vi "Dashboard Main.vi"() -> ()   [LabVIEW 2017]
uses:
  Common Code/Drivetrain Status Cluster.ctl
  Common Code/Drivetrain Mode.ctl
  Common Code/DT Encoder Values.ctl
  Common Code/Intake Status Cluster.ctl
  Common Code/Intake Mode.ctl
  Common Code/Intake States.ctl
  Common Code/Elevator Status Cluster.ctl
  Common Code/Elevator State.ctl
  Common Code/Elevator Mode.ctl
  Common Code/Intake PDP Info.ctl
  Common Code/Intake Presets.ctl
  Common Code/Drivetrain Settings Cluster.ctl
  Common Code/PID Gains Cluster.ctl
  Common Code/Elevator Settings Cluster.ctl
  Common Code/PID Gains.ctl
  Common Code/Climb Status Cluster.ctl
  Common Code/Dashboard Control Data.ctl
  Common Code/Robot Name.ctl
  Common Code/Dashboard Status Data.ctl
  <vilib>/Rock Robotics/WPI/Dashboard/WPI_DashboardLogging Global.vi
  <vilib>/Utility/inputDevices.llb/keyboardAcquire.vi
  Robot Code/Robot Global Data.vi
panel:
  in  "Save":bool
  in  "Load":bool
  out "DumbDashMessage":string
  in  "stop":bool
  in  "Tab Control":T1(tab)
  in  "Robot IP":string
  out "Drivetrain Status Cluster":T2 {"Gyro" scale=-180.0..180.0}
  in  "Drivetrain Settings Cluster":T5
  out "Elevator Status Cluster":T7={"Finished"=FALSE, "Elevator Power"=0.0, "Elevator State"=enum."Idle", "Elevator Mode"=enum."Manual", "Elevator Height"=0.0, "At Bottom?"=FALSE, "At Top?"=FALSE, "Scale high?"=FALSE, "PID Output"=0.0}
  in  "Elevator Settings Cluster":T10={"Ground Height"=0.0, "Switch Height"=0.0, "Scale High Height "=0.0, "Scale Low Height"=0.0, "Elevator PID Gains"={"proportional gain (Kc)"=1.0, "integral time (Ti, min)"=0.01, "derivative time (Td, min)"=0.0}, "Elevator Tolerance"=0.0, "Reset Encoders"=FALSE, "Encoder Scale"=0.0, "Max Height"=0.0, "Mid Height"=0.0, "output range"={"output high"=100.0, "output low"=-100.0}} {"Elevator PID Gains"."derivative time (Td, min)" format="%.3f"; "Elevator PID Gains"."integral time (Ti, min)" format="%.3f"; "Elevator PID Gains"."proportional gain (Kc)" format="%.3f"}
  out "Intake PDP Info":T12
  out "Intake Status Cluster":T13={"Intake Mode"=enum."Manual", "Intake States"=enum."Zero", "Intake Current Angle"=0.0, "Cube In Posession?"=FALSE, "Intake Wrist Up?"=FALSE}
  in  "Intake Presets":T16={"Idle Angle"=0.0, "Mid Angle"=0.0, "Low Angle"=0.0, "Outtake Power"=0.0, "Intake Power"=0.0, "Unstuck"=0.0, "Angle Tolerance"=0.0, "Max Angle"=0.0, "Max Current"=0.0, "Current Trip Time"=0.0, "Reset Encoder?"=FALSE, "Encoder Scale"=0.0, "PID gains"={"proportional gain (Kc)"=0.0, "integral time (Ti, min)"=0.0, "derivative time (Td, min)"=0.0}, "output range"={"output high"=100.0, "output low"=-100.0}}
  out "Climb Status Cluster":T17
  in  "TCP":refnum<k5>
  in  "Rec Mode":enum32{"Stop", "Record", "Playback"}(radio)
  # "A2"
  # "A3"
  # "Driver :\n\nA1 - \nA2 -\nA3 - \nA4 - \nA5 - \nB0 - \nB1 -\nB2 -\nB3 -\nB4 -\nB5 -\nB6 -\nB7 -\nB8 -\nB9 -\nUp -\nDown - \nLeft -\nRight -"
  # "Manipulator :\n\nA1 -  \nA2 -\nA3 - \nA4 - \nA5 - \nB0 - \nB1 -\nB2 -\nB3 -\nB4 -\nB5 -\nB6 -\nB7 -\nB8 -\nB9 - \nUp -\nDown - \nLeft -\nRight -"
  # "B4"
  # "B5"
  # "B6"
  # "B7"
  # "B3"
  # "U"
  # "B2"
  # "B1"
  # "L"
  # "R"
  # "A5"
  # "A1"
  # "B0"
  # "D"
  # "A0"
  # "A4"
  # "B8"
  # "B9"
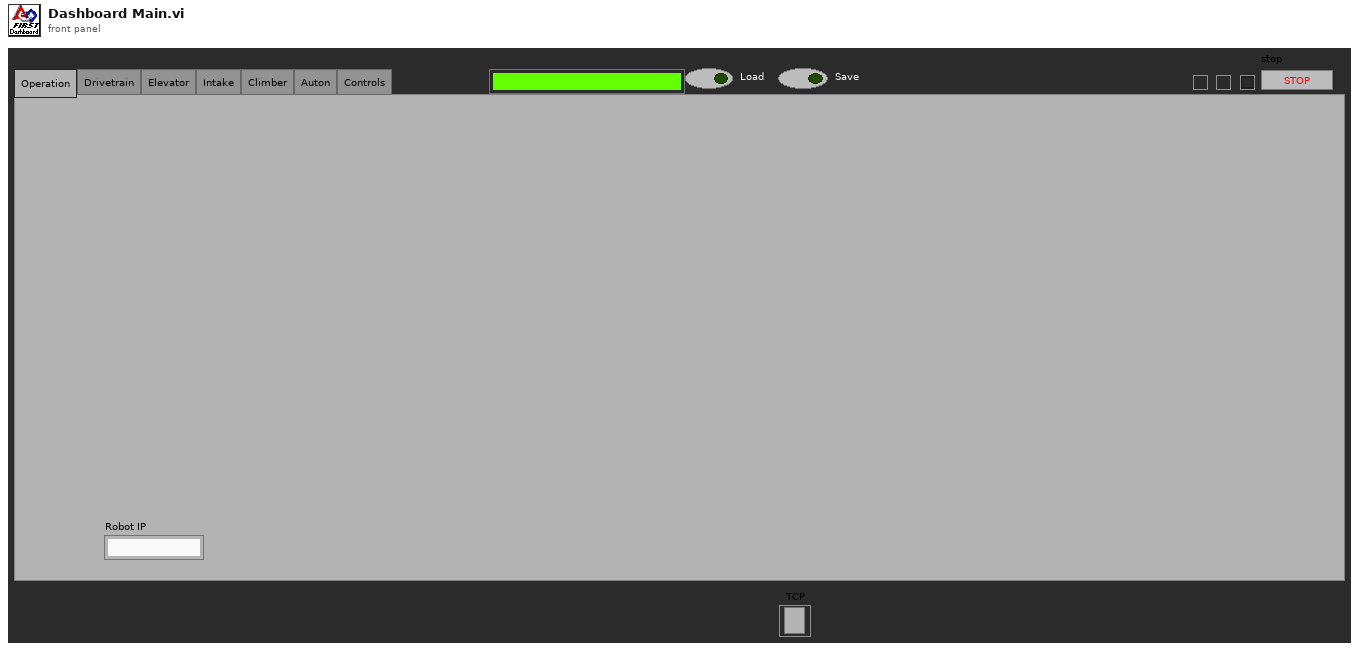
[diagram p1: front panel]
types:
  T1 = enum32{"Operation", "Drivetrain", "Elevator", "Intake", "Climber", "Auton", "Controls"}
  T2 = typedef "Drivetrain Status Cluster.ctl" = cluster{"Throttle (Y)":dbl, "Steer (X)":dbl, "Drivetrain Mode":T3, "Brake?":bool, "Distance Drive Complete?":bool, "PID Drive Complete?":bool, "Creep Mode?":bool, "Gyro Steer Complete?":bool, "Gyro":dbl, "X Max Output":dbl, "X Min Output":dbl, "Y Max Output ":dbl, "Y Min Output":dbl, "Heading Target":dbl, "Distance Target":dbl, "Gear 2":bool, "Drivetrain Encoder Values":T4}
  T3 = typedef "Drivetrain Mode.ctl" = enum16{"Manual", "Gyro Steer", "PID Drive", "Distance Drive", "Autonomous"}
  T4 = typedef "DT Encoder Values.ctl" = cluster{"Left Encoder":cluster{"Distance":dbl, "Speed":dbl, "Tick":dbl}, "Right Encoder":cluster{"Distance":dbl, "Speed":dbl, "Tick":dbl}}
  T5 = typedef "Drivetrain Settings Cluster.ctl" = cluster{"Gyro Steer PID Gains":T6, "Distance Drive PID Gains":T6, "Drive Tolerance":dbl, "Gyro Tolerance":dbl, "Gyro Output":dbl, "Distance Output":dbl, "Y Power Multiplier":dbl, "Turn Power Multiplier":dbl, "Creep Rate":dbl, "Constant Power":bool, "DT Mode Modifier":enum16{"None, Default", "Cube", "Square"}, "Left Encoder Tick Constant":dbl, "Right Encoder Tick Constant":dbl, "Shift Speed":dbl}
  T6 = typedef "PID Gains Cluster.ctl" = cluster{"Integral Time":dbl, "Proportional Gain":dbl, "Derivative Time":dbl}
  T7 = typedef "Elevator Status Cluster.ctl" = cluster{"Finished":bool, "Elevator Power":dbl, "Elevator State":T8, "Elevator Mode":T9, "Elevator Height":dbl, "At Bottom?":bool, "At Top?":bool, "Scale high?":bool, "PID Output":dbl}
  T8 = typedef "Elevator State.ctl" = enum16{"Idle", "Ground", "Mid", "Scale", "Switch"}
  T9 = typedef "Elevator Mode.ctl" = enum16{"Semi Auto", "Manual", "Auto"}
  T10 = typedef "Elevator Settings Cluster.ctl" = cluster{"Ground Height":dbl, "Switch Height":dbl, "Scale High Height ":dbl, "Scale Low Height":dbl, "Elevator PID Gains":T11, "Elevator Tolerance":dbl, "Reset Encoders":bool, "Encoder Scale":dbl, "Max Height":dbl, "Mid Height":dbl, "output range":cluster{"output high":dbl, "output low":dbl}}
  T11 = typedef "PID Gains.ctl" = cluster{"proportional gain (Kc)":dbl, "integral time (Ti, min)":dbl, "derivative time (Td, min)":dbl}
  T12 = typedef "Intake PDP Info.ctl" = cluster{"Voltage Percent Output":dbl, "Output Voltage":dbl, "Bus Voltage":dbl, "Device ID":dbl, "Output Current":dbl, "Sensor Velocity":dbl, "Sensor Position":dbl, "Pulse Width Position":dbl, "Pulse Width Velocity":dbl, "Temperature":dbl, "Inverted?":bool}
  T13 = typedef "Intake Status Cluster.ctl" = cluster{"Intake Mode":T14, "Intake States":T15, "Intake Current Angle":dbl, "Cube In Posession?":bool, "Intake Wrist Up?":bool}
  T14 = typedef "Intake Mode.ctl" = enum16{"Auto", "Semi Auto", "Manual"}
  T15 = typedef "Intake States.ctl" = enum16{"Zero", "Override Angle", "Idle", "Drop Mid", "Drop Low", "Outtake", "Intake"}
  T16 = typedef "Intake Presets.ctl" = cluster{"Idle Angle":dbl, "Mid Angle":dbl, "Low Angle":dbl, "Outtake Power":dbl, "Intake Power":dbl, "Unstuck":dbl, "Angle Tolerance":dbl, "Max Angle":dbl, "Max Current":dbl, "Current Trip Time":dbl, "Reset Encoder?":bool, "Encoder Scale":dbl, "PID gains":cluster{"proportional gain (Kc)":dbl, "integral time (Ti, min)":dbl, "derivative time (Td, min)":dbl}, "output range":cluster{"output high":dbl, "output low":dbl}}
  T17 = typedef "Climb Status Cluster.ctl" = cluster{"Climb":bool, "Time Remaining":dbl, "Button Pressed":bool}
  T18 = enum32{"Drive", "Camera", "Basic", "Custom", "Test", "Commands", "Checklist", "Variables"}
  T19 = cluster{"IDs":cluster{"RPC field ID":u16, "Unique ID":u16}, "String":string}
  T20 = typedef "Dashboard Control Data.ctl" = cluster{"Drivetrain Settings Cluster":T5, "Intake Presets":T16, "Elevator Settings Cluster":T10, "Auto Mode?":bool}
  T21 = enum16{"0", "1", "2", "3", "4", "5", "6", "7", "8", "9", "A", "B", "C", "D", "E", "F", "G", "H", "I", "J", "K", "L", "M", "N", "O", "P", "Q", "R", "S", "T", "U", "V", "W", "X", "Y", "Z", "F1", "F2", "F3", "F4", "F5", "F6", "F7", "F8", "F9", "F10", "F11", "F12", "F13", "F14", "F15", "ADD", "BACK", "BACKSLASH", "CAPITAL", "COMMA", "DECIMAL", "DELETE", "DIVIDE", "DOWN", "END", "EQUALS", "ESCAPE", "GRAVE (`)", "HOME", "INSERT", "LBRACKET", "LCONTROL", "LEFT", "L ALT", "LSHIFT", "LWIN", "MINUS", "MULTIPLY", "NEXT", "NUMLOCK", "NUMPAD_0", "NUMPAD_1", "NUMPAD_2", "NUMPAD_3", "NUMPAD_4", "NUMPAD_5", "NUMPAD_6", "NUMPAD_7", "NUMPAD_8", "NUMPAD_9", "PAUSE", "PERIOD", "PRIOR (PG UP)", "RBRACKET", "RCONTROL", "RETURN", "RIGHT", "R ALT", "RSHIFT", "RWIN", "SCROLL", "SEMICOLON", "SLASH", "SPACE", "SUBTRACT", "TAB", "UP", "ENTER (num pad)", "' (quote)"}
  T22 = enum16{"0", "1", "2", "3", "4", "5", "6", "7", "8", "9", "A", "B", "C", "D", "E", "F", "G", "H", "I", "J", "K", "L", "M", "N", "O", "P", "Q", "R", "S", "T", "U", "V", "W", "X", "Y", "Z", "F1", "F2", "F3", "F4", "F5", "F6", "F7", "F8", "F9", "F10", "F11", "F12", "F13", "F14", "F15", "ADD", "BACK", "BACKSLASH", "CAPITAL", "COMMA", "DECIMAL", "DELETE", "DIVIDE", "DOWN", "END", "EQUALS", "ESCAPE", "GRAVE (`)", "HOME", "INSERT", "LBRACKET", "LCONTROL", "LEFT", "L ALT", "LSHIFT", "LWIN", "MINUS", "MULTIPLY", "NEXT", "NUMLOCK", "NUMPAD_0", "NUMPAD_1", "NUMPAD_2", "NUMPAD_3", "NUMPAD_4", "NUMPAD_5", "NUMPAD_6", "NUMPAD_7", "NUMPAD_8", "NUMPAD_9", "PAUSE", "PERIOD", "PRIOR (PG UP)", "RBRACKET", "RCONTROL", "RETURN", "RIGHT", "R ALT", "RSHIFT", "RWIN", "SCROLL", "SEMICOLON", "SLASH", "SPACE", "SUBTRACT", "TAB", "UP", "ENTER (num pad)", "' (quote)"}[]
  T23 = typedef "Dashboard Status Data.ctl" = cluster{"Elevator Status Cluster":T7, "Drivetrain Status Cluster":T2, "Intake Status Cluster":T13, "Climb Status Cluster":T17, "Intake PDP Info":T12}
  T24 = cluster{"Error Strings":string, "Disable Counts":cluster{u16, u16}, "Rail Faults":cluster{u16, u16, u16}, "Robot IP":string, "Mode":u8, "Event Info":cluster{"Name":string, "Type":u8, "Number":u16, "Replay":u8}}
  T25 = cluster{"Storage":cluster{"Disk Free":u64, "RAM Block":u32, "RAM free":u32}, "CPU Utilization":cluster{"CPU % ISR":sgl, "CPU % Time Crit":sgl, "CPU % Timed Str":sgl, "CPU % High":sgl, "CPU % Above":sgl, "CPU % Normal":sgl, "CPU % Low":sgl}, "CAN":cluster{"% Bus Utilization":sgl, "Bus Off Cnt":u32, "TX_FIFO Full Cnt":u32, "Receive Error Cnt":u8, "Transmit Error Cnt":u8}, "HID":cluster{"HID Outputs":u32, "Rumble Low":u16, "Rumble High":u16}[]}
  T26 = cluster{"Status bits":cluster{"Test Mode":bool, "Autonomous":bool, "Enabled":bool, "Code Start":bool, "Brownout":bool, "Reserved 2":bool, "Reserved 3":bool, "E-Stop":bool}, "Code Trace":cluster{"Disabled":bool, "TeleOp":bool, "Auto":bool, "Test":bool}, "Controller Type":enum16{"unknown", "cRIO", "roboRio"}, "Code?":enum16{"unknown", "noCode", "code"}, "Battery V":dbl}
  T27 = cluster{"Control Bits":cluster{"TestMode":bool, "Autonomous":bool, "Enabled":bool, "FMS Present":bool, bool, bool, bool, "E-Stop":bool}, "Team Station ":u8, "Countdown":sgl, "Joystick Values":cluster{"Axes":dbl[], "Buttons":bool[], "POVs":i16[]}[]}
  T28 = typedef "DumbDash Control.ctl" = cluster{"Name":string, "Ref":refnum<vi>, "Type":T29}
  T29 = typedef "DumbDash Control Type.ctl" = enum16{"Invalid", "Number", "Boolean", "String"}
  T30 = cluster{"Image Size":bool, "Image Type":bool, "Pixel Value":bool, "ROI Information":bool, "Zoom Factor":bool}
  T31 = typedef "Robot Name.ctl" = u16
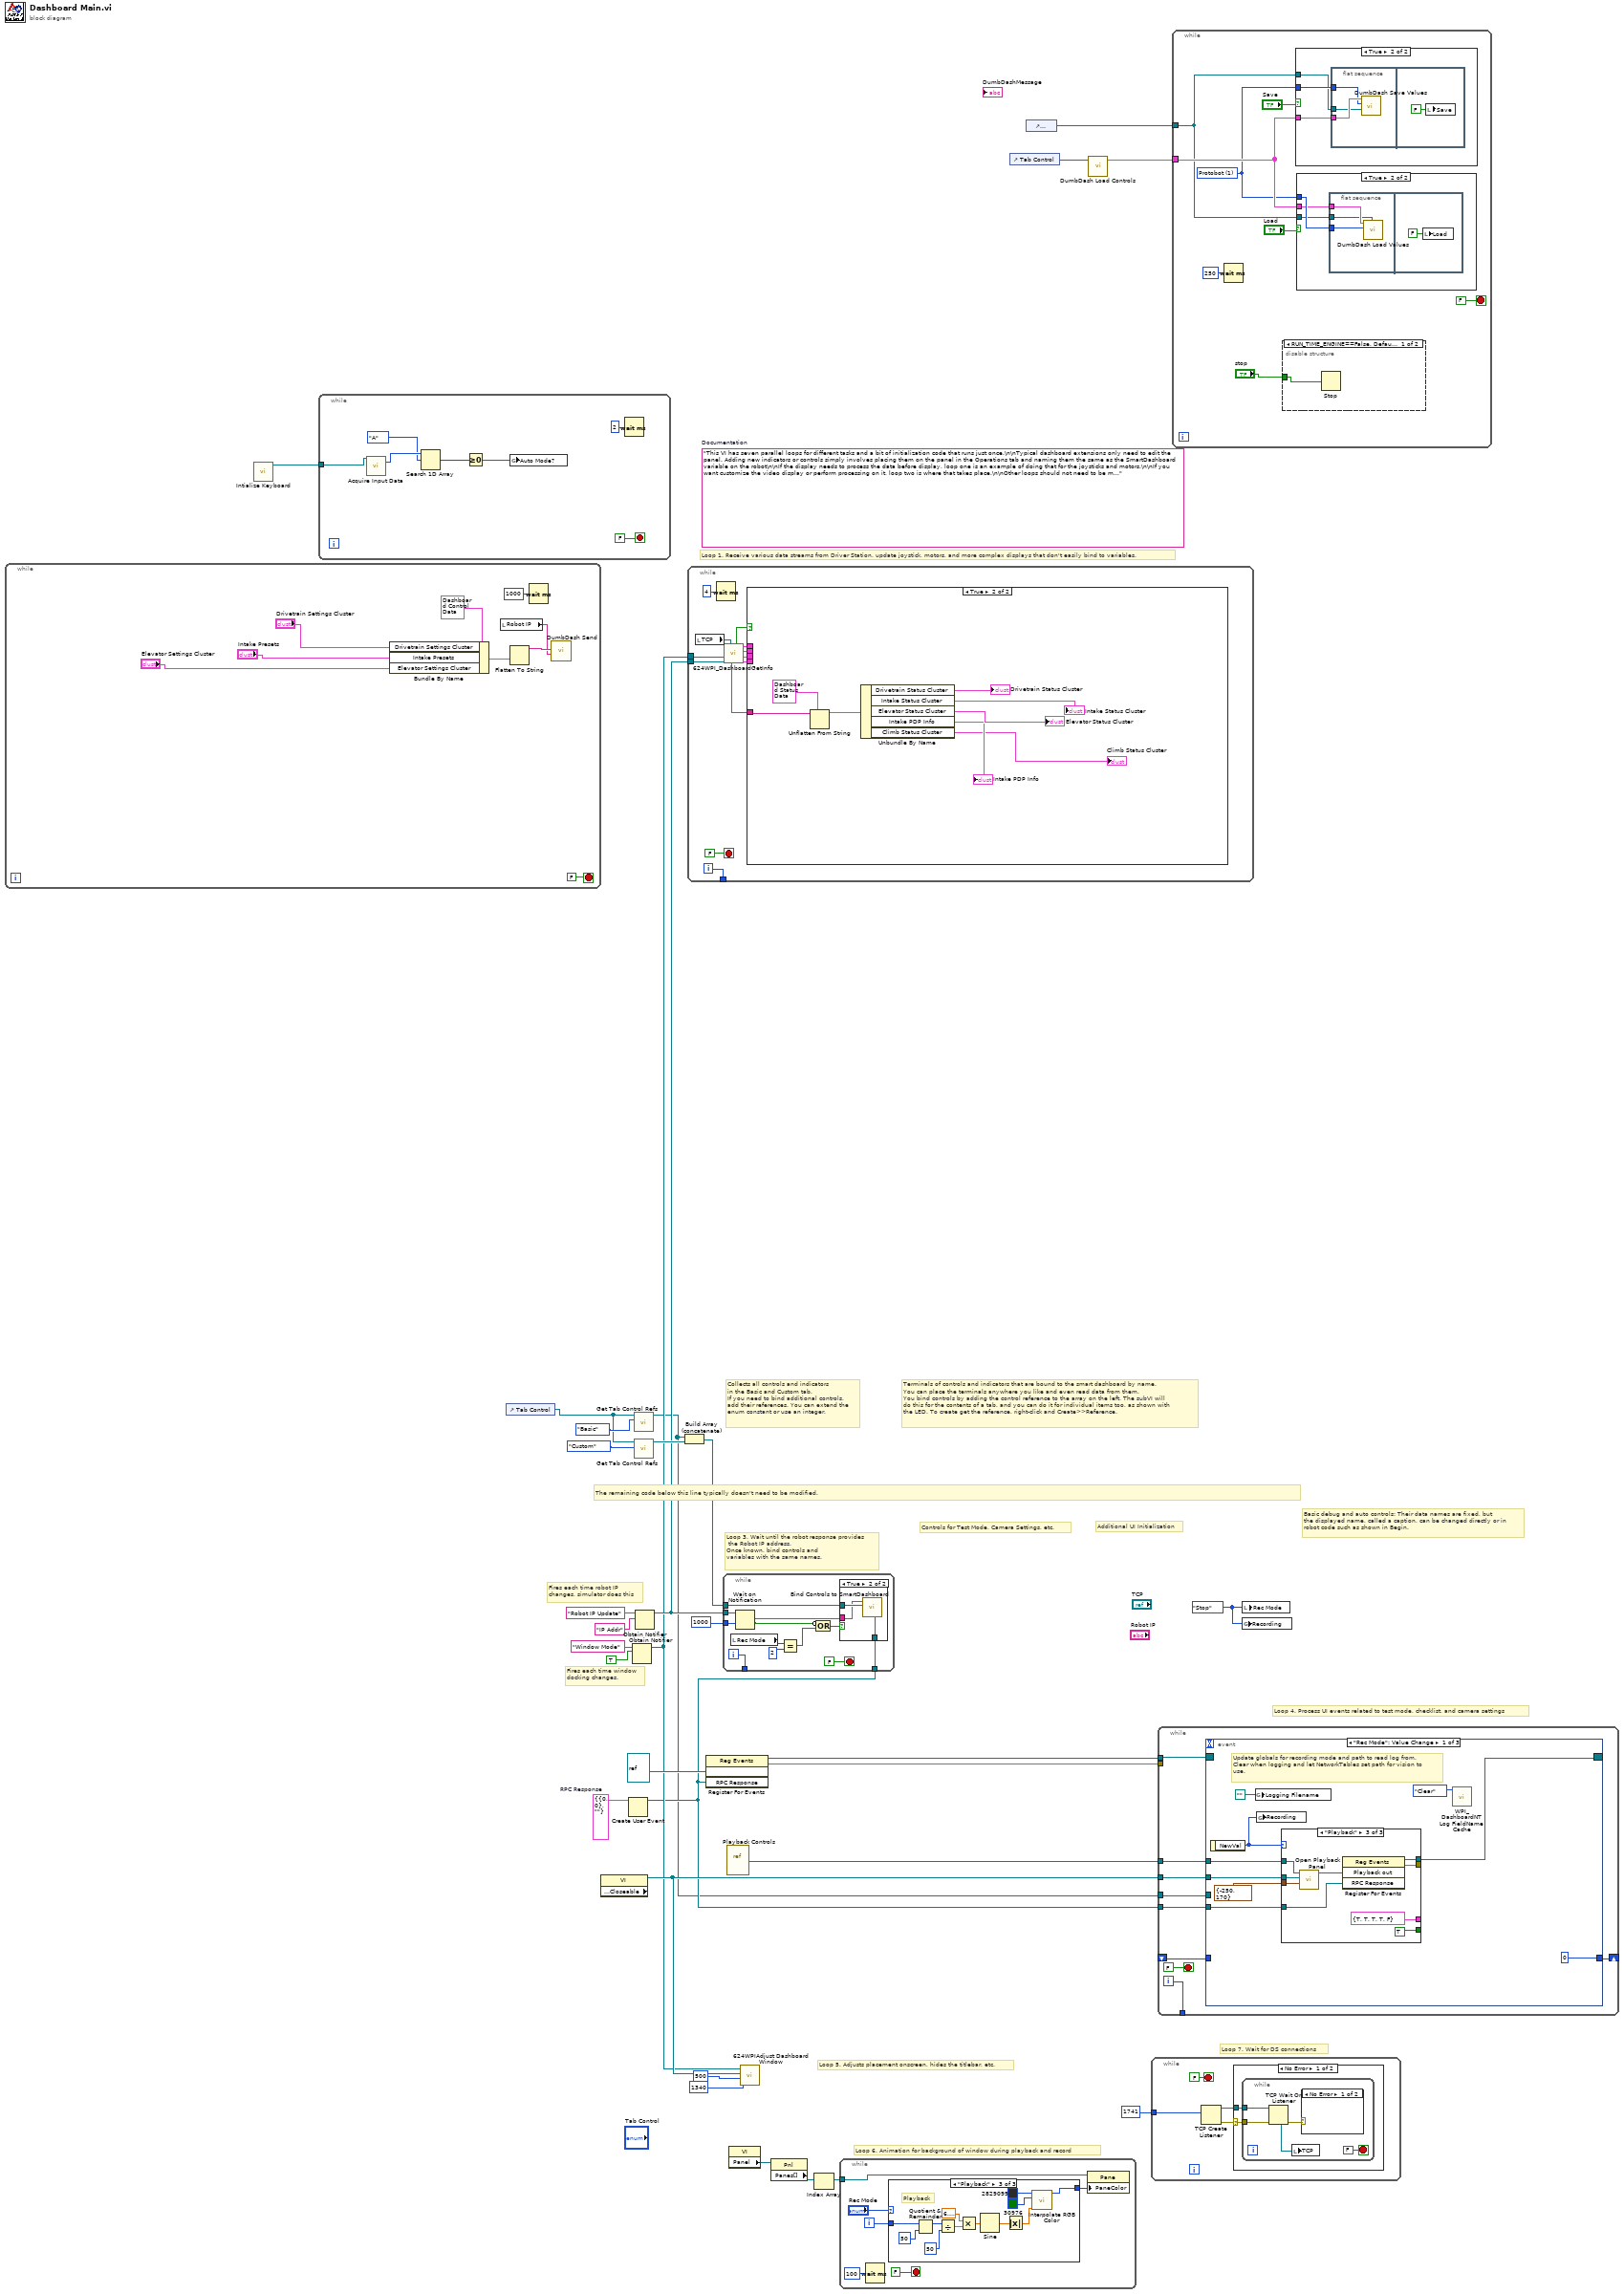
[diagram p0: block diagram]
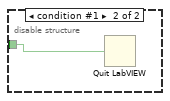
[diagram p2: hidden frame]
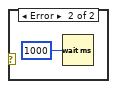
[diagram p5: hidden frame]
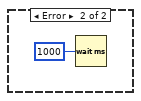
[diagram p6: hidden frame]
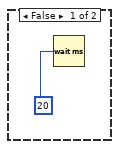
[diagram p7: hidden frame]
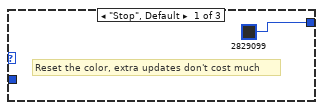
[diagram p8: hidden frame]
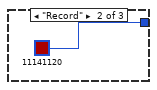
[diagram p9: hidden frame]
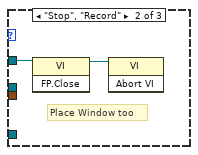
[diagram p12: hidden frame]
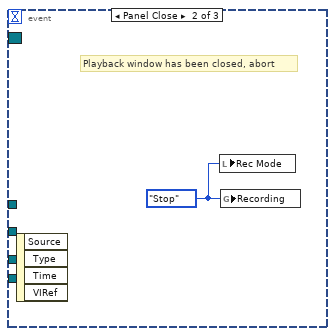
[diagram p13: hidden frame]
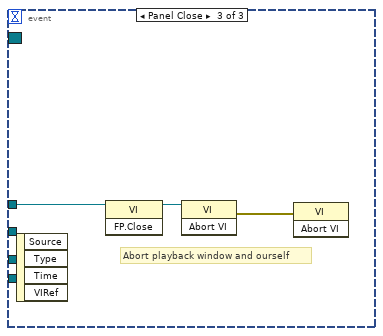
[diagram p14: hidden frame]
diagram:
  w12 = T19 {"IDs"={"RPC field ID"=0, "Unique ID"=0}, "String"=""}  # RPC Response
  w19 = enum32{"Stop", "Record", "Playback"}."Stop" ("Rec Mode")
  (unwired) "This VI has seven parallel loops for different tasks and a bit of initialization code that runs just once.\n\nTypical dashboard extensions only need to edit the panel. Adding new indicators or controls simply involves placing them on the panel in the Operations tab and naming them the same as the SmartDashboard variable on the robot\n\nIf the display needs to process the data before display, loop one is an example of doing that for the joysticks and motors.\n\nIf you want customize the video display or perform processing on it, loop two is where that takes place.\n\nOther loops should not need to be modified. They are pretty standard, and document the task they perform."  # Documentation
  # "Loop 7. Wait for DS connections"
  # "Basic debug and auto controls: Their data names are fixed, but\nthe displayed name, called a caption, can be changed directly or in\nrobot code such as shown in Begin."
  # "Controls for Test Mode, Camera Settings, etc."
  # "Additional UI Initialization"
  # "Loop 6. Animation for background of window during playback and record"
  # "Fires each time robot IP\nchanges, simulator does this"
  # "Fires each time window\ndocking changes."
  # "Collects all controls and indicators\nin the Basic and Custom tab.\nIf you need to bind additional controls,\nadd their references. You can extend the\nenum constant or use an integer."
  # "The remaining code below this line typically doesn't need to be modified."
  # "Loop 4. Process UI events related to test mode, checklist, and camera settings"
  # "Terminals of controls and indicators that are bound to the smart dashboard by name.\nYou can place the terminals anywhere you like and even read data from them.\nYou bind controls by adding the control reference to the array on the left. The subVI will\ndo this for the contents of a tab, and you can do it for individual items too, as shown with\nthe LED. To create get the reference, right-click and Create>>Reference."
  # "Loop 3. Wait until the robot response provides\n the Robot IP address.\nOnce known, bind controls and\nvariables with the same names."
  # "Loop 5. Adjusts placement onscreen, hides the titlebar, etc."
  # "Loop 1. Receive various data streams from Driver Station, update joystick, motors, and more complex displays that don't easily bind to variables."
  n1 = while {
    stop <- FALSE stop-if-true
    n2 = Bundle By Name(cluster=T20 {"Drivetrain Settings Cluster"={"Gyro Steer PID Gains"={"Integral Time"=0.0, "Proportional Gain"=0.0, "Derivative Time"=0.0}, "Distance Drive PID Gains"={"Integral Time"=0.0, "Proportional Gain"=0.0, "Derivative Time"=0.0}, "Drive Tolerance"=0.0, "Gyro Tolerance"=0.0, "Gyro Output"=0.0, "Distance Output"=0.0, "Y Power Multiplier"=0.0, "Turn Power Multiplier"=0.0, "Creep Rate"=0.0, "Constant Power"=FALSE, "DT Mode Modifier"=enum."None, Default", "Left Encoder Tick Constant"=0.0, "Right Encoder Tick Constant"=0.0, "Shift Speed"=0.0}, "Intake Presets"={"Idle Angle"=0.0, "Mid Angle"=0.0, "Low Angle"=0.0, "Outtake Power"=0.0, "Intake Power"=0.0, "Unstuck"=0.0, "Angle Tolerance"=0.0, "Max Angle"=0.0, "Max Current"=0.0, "Current Trip Time"=0.0, "Reset Encoder?"=FALSE, "Encoder Scale"=0.0, "PID gains"={"proportional gain (Kc)"=0.0, "integral time (Ti, min)"=0.0, "derivative time (Td, min)"=0.0}, "output range"={"output high"=100.0, "output low"=-100.0}}, "Elevator Settings Cluster"={"Ground Height"=0.0, "Switch Height"=0.0, "Scale High Height "=0.0, "Scale Low Height"=0.0, "Elevator PID Gains"={"proportional gain (Kc)"=1.0, "integral time (Ti, min)"=0.01, "derivative time (Td, min)"=0.0}, "Elevator Tolerance"=0.0, "Reset Encoders"=FALSE, "Encoder Scale"=0.0, "Max Height"=0.0, "Mid Height"=0.0, "output range"={"output high"=0.0, "output low"=0.0}}, "Auto Mode?"=FALSE} ("Dashboard Control Data"), "Drivetrain Settings Cluster"="Drivetrain Settings Cluster", "Intake Presets"="Intake Presets", "Elevator Settings Cluster"="Elevator Settings Cluster") -> (w32:T20)
    n3 = local read "Robot IP"() -> (w36:string)
    n4 = Flatten To String(anything=w32) -> (data string=w40:string)  [unwired: 3 in, 2 out]
    n5 = Wait (ms)(milliseconds to wait=u32 1000) -> ()  [unwired: 1 out]
    n6 = call "DumbDash Send.vi"("Robot IP"=w36, "data string"=w40) -> ()  [unwired: 10 in]
  }
  n7 = call <vilib>:"Intialize Keyboard.vi"() -> ("device ID"=w1:refnum<k1>)  [unwired: 10 in, 1 out]
  n8 = while {
    tunnel: w1 -> [w47]
    stop <- FALSE stop-if-true
    n9 = call-poly <vilib>:"Acquire Input Data.vi"("device ID"=w47) -> ("keys pressed"=w46:T22)  [unwired: 16 in, 2 out]
    n10 = Search 1D Array(1D array=w46, element=T21."A" ("keyType 3")) -> (index of element=w44:i32)  [unwired: 1 in]
    n11 = Greater Or Equal To 0?(x=w44) -> (x >= 0?=w41:bool)
    n12 = global write "Robot Global Data.vi" "Auto Mode?"(w41) -> ()
    n13 = Wait (ms)(milliseconds to wait=u32 2) -> ()  [unwired: 1 out]
  }
  n14 = control-ref of="Tab Control"() -> (w4:refnum<vi>)
  n15 = property class="VI" props=["Front Panel.Closeable"]() -> (reference out=w18:refnum<vi>)  [unwired: 2 in, 2 out]
  n16 = Create User Event(user event datatype=w12) -> (user event=w11:refnum<user-event>)  [unwired: 1 in, 1 out]
  n17 = Obtain Notifier(name (unnamed)="Window Mode", notification data type=TRUE) -> (notifier out=w14:refnum<notifier>)  [unwired: 2 in, 2 out]
  n18 = call <vilib>:"Get Tab Control Refs.vi"("Page Index"=T18."Basic" ("Dashboard Tab"), "TabControl in"=w4) -> ("ControlsOnPage"=w10:refnum<vi>[])  [unwired: 9 in]
  n19 = call <vilib>:"Get Tab Control Refs.vi"("Page Index"=T18."Custom" ("Dashboard Tab"), "TabControl in"=w4) -> ("ControlsOnPage"=w17:refnum<vi>[])  [unwired: 9 in]
  n20 = Obtain Notifier(name (unnamed)="Robot IP Update", notification data type="IP Addr" ("name (unnamed)")) -> (notifier out=w15:refnum<notifier>)  [unwired: 2 in, 2 out]
  n21 = Build Array (concatenate)(w10, w17) -> (w16:refnum<vi>[])
  n22 = while {
    tunnel: [w58] -> _
    tunnel: w15 -> [w56]
    tunnel: w14 -> [w57]
    i -> [w58]
    stop <- FALSE stop-if-true
    n23 = local read "TCP"() -> (w55:refnum<k5>)
    n24 = Wait (ms)(milliseconds to wait=u32 4) -> ()  [unwired: 1 out]
    n25 = call "624WPI_DashboardGetInfo.vi"("Binding Refnum"=w56, "Window Mode Notifier"=w57, "TCP Cnx"=w55) -> ("Power and Errors"=w50:T24, "Robot Metrics"=w51:T25, "Status Info"=w52:T26, "Control Info"=w53:T27, "Process?"=w54:bool, "Custom Dashboard Data"=w49:string)  [unwired: 2 in, 1 out]
    n26 = case shown="True" w54 {
      tunnel: w53 -> [_ _]
      tunnel: w52 -> [_ _]
      tunnel: w51 -> [_ _]
      tunnel: w50 -> [_ _]
      tunnel: w49 -> [_ w68]
      frame False {
        n27 = Wait (ms)(milliseconds to wait=u32 20) -> ()  [unwired: 1 out]
      }
      frame True {
        n28 = Unflatten From String(type=T23 {"Elevator Status Cluster"={"Finished"=FALSE, "Elevator Power"=0.0, "Elevator State"=enum."Idle", "Elevator Mode"=enum."Manual", "Elevator Height"=0.0, "At Bottom?"=FALSE, "At Top?"=FALSE, "Scale high?"=FALSE, "PID Output"=0.0}, "Drivetrain Status Cluster"={"Throttle (Y)"=0.0, "Steer (X)"=0.0, "Drivetrain Mode"=enum."Manual", "Brake?"=FALSE, "Distance Drive Complete?"=FALSE, "PID Drive Complete?"=FALSE, "Creep Mode?"=FALSE, "Gyro Steer Complete?"=FALSE, "Gyro"=0.0, "X Max Output"=0.0, "X Min Output"=0.0, "Y Max Output "=0.0, "Y Min Output"=0.0, "Heading Target"=0.0, "Distance Target"=0.0, "Gear 2"=FALSE, "Drivetrain Encoder Values"={"Left Encoder"={"Distance"=0.0, "Speed"=0.0, "Tick"=0.0}, "Right Encoder"={"Distance"=0.0, "Speed"=0.0, "Tick"=0.0}}}, "Intake Status Cluster"={"Intake Mode"=enum."Auto", "Intake States"=enum."Zero", "Intake Current Angle"=0.0, "Cube In Posession?"=FALSE, "Intake Wrist Up?"=FALSE}, "Climb Status Cluster"={"Climb"=FALSE, "Time Remaining"=0.0, "Button Pressed"=FALSE}, "Intake PDP Info"={"Voltage Percent Output"=0.0, "Output Voltage"=0.0, "Bus Voltage"=0.0, "Device ID"=0.0, "Output Current"=0.0, "Sensor Velocity"=0.0, "Sensor Position"=0.0, "Pulse Width Position"=0.0, "Pulse Width Velocity"=0.0, "Temperature"=0.0, "Inverted?"=FALSE}} ("Dashboard Status Data"), binary string=w68) -> (value=w66:T23)  [unwired: 3 in, 2 out]
        n29 = Unbundle By Name(w66) -> ("Drivetrain Status Cluster"=→"Drivetrain Status Cluster":T2, "Intake Status Cluster"=→"Intake Status Cluster":T13, "Elevator Status Cluster"=→"Elevator Status Cluster":T7, "Intake PDP Info"=→"Intake PDP Info":T12, "Climb Status Cluster"=→"Climb Status Cluster":T17)
      }
    }
  }
  n30 = register-events(refnum<vi> refnum, w11) -> (reference out=w23:refnum<event-registration>, error out=w22:errorcluster)  [unwired: 2 in]
  n31 = while {
    tunnel: w16 -> [w80]
    tunnel: w15 -> [w78]
    tunnel: [w76] -> _
    tunnel: u32 1000 ("milliseconds to wait") -> [w75]
    tunnel: w11 -> [w69]
    i -> [w76]
    stop <- FALSE stop-if-true
    n32 = local read "Rec Mode"() -> (w71:enum32{"Stop", "Record", "Playback"})
    n33 = Wait on Notification(notifier=w78, timeout in ms (-1)=w75) -> (notification=w77:string, timed out?=w73:bool)  [unwired: 2 in, 2 out]
    n34 = Equal?(x=w71, y=u16 2 ("Rec Mode")) -> (x = y?=w72:bool)
    n35 = Compound Arithmetic op=OR(invert w73, w72) -> (w74:bool)
    n36 = case shown="True" w74 {
      tunnel: w80 -> [_ w83]
      tunnel: w77 -> [_ w82]
      tunnel: w69 -> [_ w81]
      frame False {
      }
      frame True {
        n37 = call <vilib>:"Bind Controls to SmartDashboard.vi"("RPC ref"=w81, "Bound Control Refs"=w83, "Server IP Address"=w82) -> ()  [unwired: 9 in]
      }
    }
  }
  n38 = vi-ref "Playback Controls.vi"() -> (w24:refnum<vi>)
  n39 = property class="VI"() -> ("Panel"=w26:refnum<vi>)  [unwired: 2 in, 2 out]
  n40 = call "624WPIAdjust Dashboard Window.vi"("Width"=i16 1340, "Height"=i16 500, "VI"=w18, "Notifier in"=w14) -> ()  [unwired: 8 in]
  n41 = property class="Pnl"(reference=w26) -> ("Panes[]"=w27:refnum<vi>[])  [unwired: 1 in, 2 out]
  n42 = Index Array(array=w27) -> (element=w25:refnum<vi>)  [unwired: 1 in]
  n43 = while {
    tunnel: w25 -> [w85]
    i -> [w88]
    stop <- FALSE stop-if-true
    n44 = Wait (ms)(milliseconds to wait=u32 100) -> ()  [unwired: 1 out]
    n45 = case shown="\"Playback\"" "Rec Mode" {
      tunnel: w88 -> [_ _ w103]
      tunnel: [u32 2829099 ("Base Color") u32 11141120 ("Target Color") w92] -> w84
      frame "Stop", Default {
        # "Reset the color, extra updates don't cost much"
      }
      frame "Record" {
      }
      frame "Playback" {
        # "Playback"
        n46 = Quotient & Remainder(x=w103, y=u32 50 ("milliseconds to wait")) -> (x-y*floor(x/y)=w99:u32)  [unwired: 1 out]
        n47 = Divide(x=w99, y=u32 50 ("milliseconds to wait")) -> (x/y=w96:dbl)
        n48 = Multiply(x=6.283185307179586, y=w96) -> (x*y=w101:dbl)
        n49 = Sine(x=w101) -> (sin(x)=w100:dbl)
        n50 = Absolute Value(x=w100) -> (abs(x)=w93:dbl)
        n51 = call "Interpolate RGB Color.vi"("Proportion"=w93, "Target Color"=u32 30976, "Base Color"=u32 2829099) -> ("Result Color"=w92:u32)  [unwired: 8 in]
      }
    }
    n52 = property class="Pane"(reference=w85, "PaneColor"=w84) -> ()  [unwired: 1 in, 2 out]
  }
  n53 = control-ref of="Tab Control"() -> (w3:refnum<vi>)
  n54 = control-ref of="DumbDashMessage"() -> (w5:refnum<vi>)
  n55 = call "DumbDash Load Controls.vi"("TabControl in"=w3) -> ("Array"=w6:T28[])  [unwired: 10 in]
  n56 = while {
    tunnel: u16 1741 ("timeout ms (25000)") -> [w105]
    stop <- FALSE stop-if-true
    n57 = TCP Create Listener(10:w105) -> (0:w104:errorcluster, 3:w106:refnum<k5>)  [unwired: 4 in, 1 out]
    n58 = case shown="No Error" w104 {
      selector: w104 -> [w108 _]
      tunnel: w106 -> [w109 _]
      frame No Error {
        n59 = while {
          tunnel: w109 -> [w113]
          tunnel: w108 -> [w112]
          stop <- FALSE stop-if-true
          n60 = TCP Wait On Listener(8:w112, 11:w113) -> (0:w114:errorcluster, 4:w110:refnum<k5>)  [unwired: 2 in, 3 out]
          n61 = local write "TCP"(w110) -> ()
          n62 = case shown="No Error" w114 {
            frame No Error {
            }
            frame Error {
              n63 = Wait (ms)(milliseconds to wait=u32 1000) -> ()  [unwired: 1 out]
            }
          }
        }
      }
      frame Error {
        n64 = Wait (ms)(milliseconds to wait=u32 1000) -> ()  [unwired: 1 out]
      }
    }
  }
  n65 = while {
    tunnel: [w124] -> _
    tunnel: w24 -> [w123]
    tunnel: w23 -> [w122]
    tunnel: w22 -> [_]
    tunnel: w18 -> [w121]
    tunnel: w11 -> [w120]
    shift-right: [w119] -> _
    shift-left: _ -> [w118]
    tunnel: w10 -> [w117]
    i -> [w124]
    stop <- FALSE stop-if-true
    n66 = event shown="[0] \"Rec Mode\": Value Change" {
      selector: w122 -> [_ _ _]
      dyn-events: [w131 _ _] -> _
      timeout: _ -> [_ _ _]
      tunnel: w123 -> [w133 _ w149]
      tunnel: w121 -> [w129 _ _]
      tunnel: w120 -> [w127 _ _]
      tunnel: [0 _ _] -> w119
      tunnel: w118 -> [_ _ _]
      tunnel: w117 -> [_ _ _]
      event "Rec Mode": Value Change {
        # "Update globals for recording mode and path to read log from.\nClear when logging and let NetworkTables set path for vision to\nuse."
        n67 = event-data() -> ("NewVal"=w134:enum32{"Stop", "Record", "Playback"})  [unwired: 1 in]
        n68 = global write "WPI_DashboardLogging Global.vi" "Logging Filename"(path "") -> ()
        n69 = global write "WPI_DashboardLogging Global.vi" "Recording"(w134) -> ()
        n70 = case shown="\"Playback\"" w134 {
          tunnel: w133 -> [_ w136 w145]
          tunnel: [_ _ w144] -> w131
          tunnel: [_ _ w143] -> _
          tunnel: w129 -> [_ _ w141]
          tunnel: cluster{i32, i32} {-250, 170} -> [_ _ w140]
          tunnel: [_ _ T30 {"Image Size"=TRUE, "Image Type"=TRUE, "Pixel Value"=TRUE, "ROI Information"=TRUE, "Zoom Factor"=FALSE} ("Image Information Shown:All Elements")] -> _
          tunnel: [_ _ TRUE ("Zoom Factor")] -> _
          tunnel: w127 -> [_ _ w137]
          frame Default {
          }
          frame "Stop", "Record" {
            # "Place Window too"
            n71 = invoke class="VI" method="FP.Close"(reference=w136) -> (reference out=w135:refnum<vi>)  [unwired: 2 in, 2 out]
            n72 = invoke class="VI" method="Abort VI"(reference=w135) -> ()  [unwired: 2 in, 3 out]
          }
          frame "Playback" {
            n73 = call "Open Playback Panel.vi"("Offset"=w140, "DB VI Ref"=w141, "Playback in"=w145) -> ("Playback out"=w142:refnum<vi>)  [unwired: 8 in]
            n74 = register-events(w142, w137) -> (reference out=w144:refnum<event-registration>, error out=w143:errorcluster)  [unwired: 2 in]
          }
        }
        n75 = call <vilib>:"WPI_DashboardNT Log FieldName Cache.vi"("Operation"=enum16{"Lookup/Add", "Index", "Clear"}."Clear") -> ()  [unwired: 8 in, 3 out]
      }
      event Panel Close {
        w146 = enum32{"Stop", "Record", "Playback"}."Stop" ("Rec Mode")
        # "Playback window has been closed, abort"
        n76 = event-data() -> ()  [unwired: 1 in, 4 out]
        n77 = local write "Rec Mode"(w146) -> ()
        n78 = global write "WPI_DashboardLogging Global.vi" "Recording"(w146) -> ()
      }
      event Panel Close {
        # "Abort playback window and ourself"
        n79 = event-data() -> ()  [unwired: 1 in, 4 out]
        n80 = invoke class="VI" method="FP.Close"(reference=w149) -> (reference out=w148:refnum<vi>)  [unwired: 2 in, 2 out]
        n81 = invoke class="VI" method="Abort VI"(reference=w148) -> (error out=w147:errorcluster)  [unwired: 2 in, 2 out]
        n82 = invoke class="VI" method="Abort VI"(error in=w147) -> ()  [unwired: 2 in, 3 out]
      }
    }
  }
  n83 = while {
    tunnel: w6 -> [w154]
    tunnel: w5 -> [w152]
    stop <- FALSE stop-if-true
    w153 = T31 1 items=["Main Bot", "Protobot"] ("Robot")
    n84 = Wait (ms)(milliseconds to wait=u32 250) -> ()  [unwired: 1 out]
    n85 = disable-structure shown="RUN_TIME_ENGINE==False, Default" {
      disable-tunnel: "stop" -> [w158 w159]
      frame condition #0 (active) {
        n86 = Stop(stop? (T)=w158) -> ()
      }
      frame condition #1 {
        n87 = Quit LabVIEW(quit? (T)=w159) -> ()
      }
    }
    n88 = case shown="True" "Save" {
      tunnel: w154 -> [_ w169]
      tunnel: w153 -> [_ w168]
      tunnel: w152 -> [_ w167]
      frame False {
      }
      frame True {
        n89 = flat-sequence {
          tunnel: w169 -> [w172]
          tunnel: w168 -> [w171]
          tunnel: w167 -> [w170]
          frame #0 {
            n90 = call "DumbDash Save Values.vi"("Message Box"=w170, "Robot"=w171, "Controls In"=w172) -> ()  [unwired: 9 in]
          }
          frame #1 {
            n91 = local write "Save"(FALSE ("Save")) -> ()
          }
        }
      }
    }
    n92 = case shown="True" "Load" {
      tunnel: w154 -> [_ w161]
      tunnel: w153 -> [_ w162]
      tunnel: w152 -> [_ w160]
      frame False {
      }
      frame True {
        n93 = flat-sequence {
          tunnel: w162 -> [w165]
          tunnel: w161 -> [w164]
          tunnel: w160 -> [w163]
          frame #0 {
            n94 = call "DumbDash Load Values.vi"("Message Box"=w163, "Robot"=w165, "Controls In"=w164) -> ()  [unwired: 9 in]
          }
          frame #1 {
            n95 = local write "Load"(FALSE ("Load")) -> ()
          }
        }
      }
    }
  }
  n96 = global write "WPI_DashboardLogging Global.vi" "Recording"(w19) -> ()
  n97 = local write "Rec Mode"(w19) -> ()
